vi "Parse Response JSON.vi"(8 "error in (no error)":errorcluster, 10 "Response JSON":string, 11 "RJSONDebug in":refnum<class "RJSONDebug.lvclass">) -> (0 "error out":errorcluster, 3 "RJSONDebug out":refnum<class "RJSONDebug.lvclass">)   [LabVIEW 2022 SP3, in "obs-websocket-lv.lvlib" / "RJSONDebug.lvclass"]
uses:
  RJSONDebug.lvclass
  RJSONDebug.lvclass/RJSONDebug.ctl
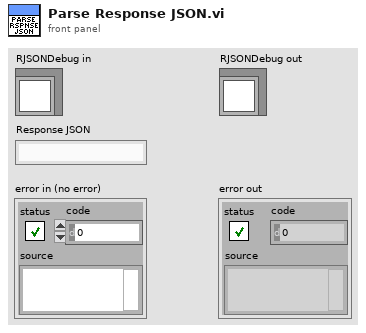
[diagram p1: front panel]
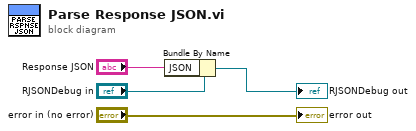
[diagram p0: block diagram]
diagram:
  n1 = Bundle By Name(cluster="RJSONDebug in", "JSON"="Response JSON") -> (→"RJSONDebug out":refnum<class "RJSONDebug.lvclass">)
  "error out" <- "error in (no error)"
